vi "ECG.vi"() -> ()   [LabVIEW 2019]
uses:
  <vilib>/addons/Biomedical/Biosignal Measurements/Biosignal Preprocessing/Biosignal Rate Extractor (Waveform).vi
  <vilib>/addons/Biomedical/NI_BMTK_Measurements.lvlib
panel:
  out "BPM":dbl
  out "R-R":dbl format="%#.6g"
  in  "stop":bool
  out "ECG":dynamicdata(graph)
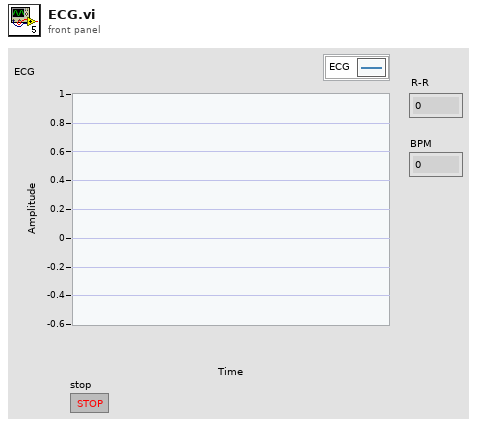
[diagram p1: front panel]
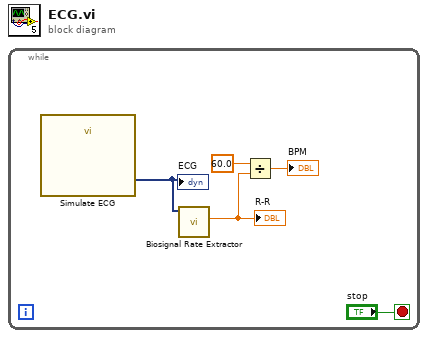
[diagram p0: block diagram]
diagram:
  n1 = while {
    stop <- "stop" stop-if-true
    n2 = call "Simulate ECG"() -> ("ECG"=w4:dynamicdata)  [unwired: 10 in, 1 out]
    "ECG" <- w4
    n3 = call-poly <vilib>:"Biosignal Rate Extractor.vi"("biosignal"=w4) -> ("mean cycle time"=w2:dbl)  [unwired: 8 in, 2 out]
    "R-R" <- w2
    n4 = Divide(x=60.0, y=w2) -> (x/y=→"BPM":dbl)
  }
